vi "Thor_GetSEtVelParam.vi"(5 "acceleration":dbl, 7 "maxVelocity":dbl, 8 "error in (no error)":errorcluster, 9 "Set Param":bool, 10 "Device In":T1, 11 "KCubeServoControl In":T2) -> (0 "error out":errorcluster, 2 "Device Out":T1, 3 "KCubeServoControl out":T2, 4 "accelerationOut":dbl, 6 "maxVelocityOut":dbl)   [LabVIEW 2020]
uses:
  Thor_KCubeServoDCRef.ctl
  E:/Norway Project/All Hardware/New Microscope/LabVIEW/ThorLabs/Thorlabs.MotionControl.Controls.dll
  Thorlabs.MotionControl.Controls.dll
  Thor_DeviceRef.ctl
  E:/Norway Project/All Hardware/New Microscope/LabVIEW/ThorLabs/ThorLabs.MotionControl.KCube.DCServoCLI.dll
  ThorLabs.MotionControl.KCube.DCServoCLI.dll
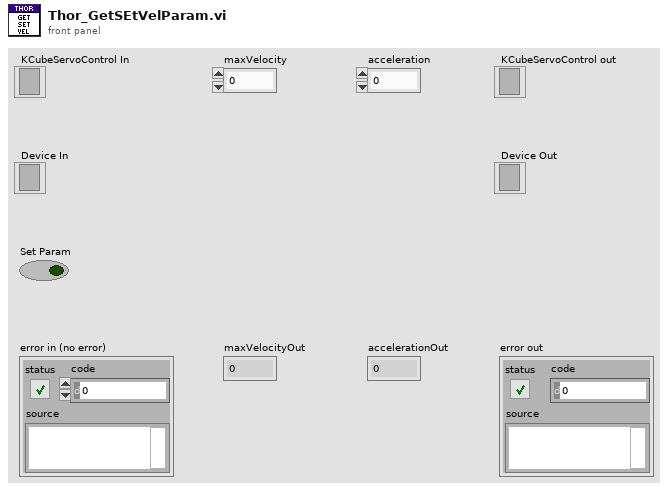
[diagram p1: front panel]
types:
  T1 = typedef "Thor_DeviceRef.ctl" = refnum<k24>
  T2 = typedef "Thor_KCubeServoDCRef.ctl" = refnum<k24>
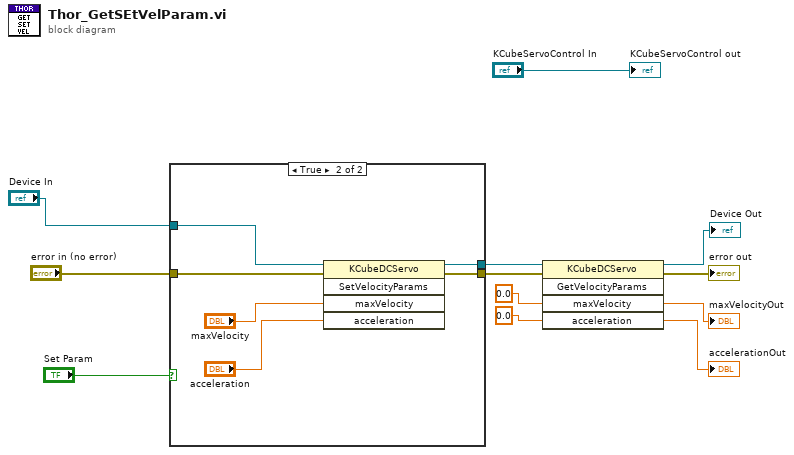
[diagram p0: block diagram]
diagram:
  n1 = case shown="True" "Set Param" {
    tunnel: "Device In" -> [w14 w20]
    tunnel: "error in (no error)" -> [w13 w19]
    tunnel: [w14 w16] -> w7
    tunnel: [w13 w15] -> w5
    frame False {
    }
    frame True {
      n2 = invoke class="KCubeDCServo" method="SetVelocityParams"(reference=w20, error in=w19, "maxVelocity"="maxVelocity", "acceleration"="acceleration") -> (reference out=w16:T1, error out=w15:errorcluster)  [unwired: 1 in, 3 out]
    }
  }
  n3 = invoke class="KCubeDCServo" method="GetVelocityParams"(reference=w7, error in=w5, "maxVelocity"=0.0, "acceleration"=0.0) -> (reference out=→"Device Out":T1, error out=→"error out":errorcluster, "maxVelocity"=→"maxVelocityOut":dbl, "acceleration"=→"accelerationOut":dbl)  [unwired: 1 in, 1 out]
  "KCubeServoControl out" <- "KCubeServoControl In"
